vi "Configure Resistor Band Visibility.vi.vi"(8 "error in (no error)":errorcluster, 9 "Number of Bands":u8=4 min=3 max=6 step=1, 11 "Color Box Refnum":refnum<vi>[](array[refnum])) -> (0 "error out":errorcluster)   [LabVIEW 2018]
doc: "Configures the visibility of the resistor band ColorBox controls on the Front Panel according to the selected number of bands.\n\nThe VI receives the <b>Number of Bands</b> and an array of <b>ColorBox Refnums</b>. It determines which resistor bands must be visible for 3-, 4-, 5-, and 6-band resistor configurations and updates the <b>Visible</b> property of each ColorBox control.\n\nThe VI only configures Front Panel visibility. It does not modify the color or value of any resistor band."
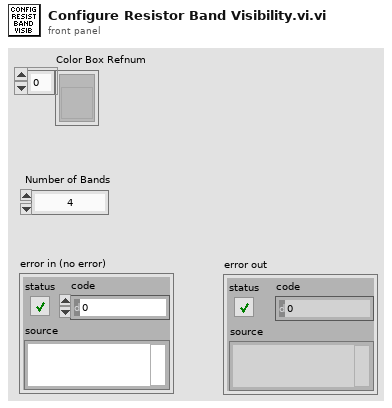
[diagram p1: front panel]
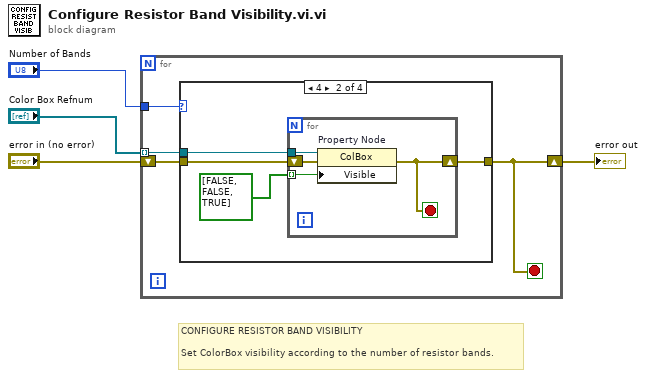
[diagram p0: block diagram]
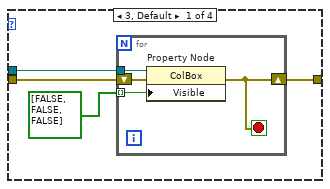
[diagram p2: hidden frame]
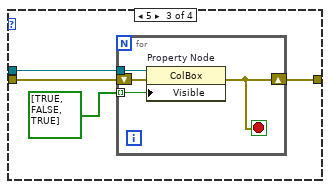
[diagram p3: hidden frame]
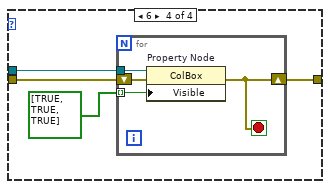
[diagram p4: hidden frame]
diagram:
  # "CONFIGURE RESISTOR BAND VISIBILITY\n\nSet ColorBox visibility according to the number of resistor bands."
  n1 = for {
    tunnel: "Number of Bands" -> [w8]
    tunnel: "Color Box Refnum" -> [w7] mode=indexing
    shift-right: [w5] -> w4
    shift-left: "error in (no error)" -> [w6]
    stop <- w5 stop-if-true
    n2 = case shown="4" w8 {
      tunnel: w7 -> [w12 w20 w28 w36]
      tunnel: [w10 w17 w25 w33] -> w5
      tunnel: w6 -> [w9 w18 w26 w34]
      frame 3, Default {
        n3 = for {
          tunnel: w12 -> [w16]
          tunnel: bool[] [FALSE, FALSE, FALSE] -> [w15] mode=indexing
          shift-right: [w13] -> w10
          shift-left: w9 -> [w14]
          stop <- w13 stop-if-true
          n4 = property on="Property Node" class="ColBox"(reference=w16, error in=w14, "Visible"=w15) -> (error out=w13:errorcluster)  [unwired: 1 out]
        }
      }
      frame 4 {
        n5 = for {
          tunnel: w20 -> [w24]
          tunnel: bool[] [FALSE, FALSE, TRUE] -> [w23] mode=indexing
          shift-right: [w21] -> w17
          shift-left: w18 -> [w22]
          stop <- w21 stop-if-true
          n6 = property on="Property Node" class="ColBox"(reference=w24, error in=w22, "Visible"=w23) -> (error out=w21:errorcluster)  [unwired: 1 out]
        }
      }
      frame 5 {
        n7 = for {
          tunnel: w28 -> [w32]
          tunnel: bool[] [TRUE, FALSE, TRUE] -> [w31] mode=indexing
          shift-right: [w29] -> w25
          shift-left: w26 -> [w30]
          stop <- w29 stop-if-true
          n8 = property on="Property Node" class="ColBox"(reference=w32, error in=w30, "Visible"=w31) -> (error out=w29:errorcluster)  [unwired: 1 out]
        }
      }
      frame 6 {
        n9 = for {
          tunnel: w36 -> [w40]
          tunnel: bool[] [TRUE, TRUE, TRUE] -> [w39] mode=indexing
          shift-right: [w37] -> w33
          shift-left: w34 -> [w38]
          stop <- w37 stop-if-true
          n10 = property on="Property Node" class="ColBox"(reference=w40, error in=w38, "Visible"=w39) -> (error out=w37:errorcluster)  [unwired: 1 out]
        }
      }
    }
  }
  "error out" <- w4
